vi "Cmd.Trigger.vi"(6 "Timeout [ms] (1000)":i32=1000, 8 "error in":errorcluster, 10 "TriggerNo":T1 items=["1"=1, "2"=2, "3"=3, "4"=4, "ALL"=5], 11 "cID in":refnum<k5>) -> (0 "error out":errorcluster, 1 "debug":string, 3 "cID out":refnum<k5>)   [LabVIEW 2016]
uses:
  controls/TriggerNo.ctl
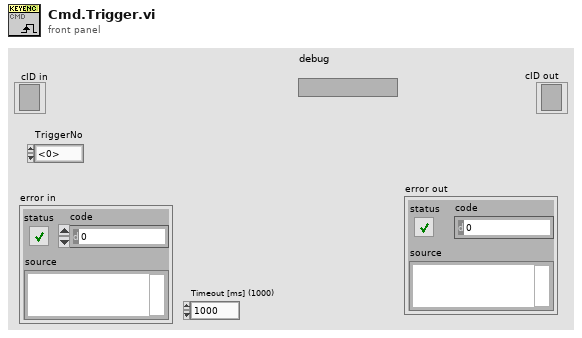
[diagram p1: front panel]
types:
  T1 = typedef "TriggerNo.ctl" = u8
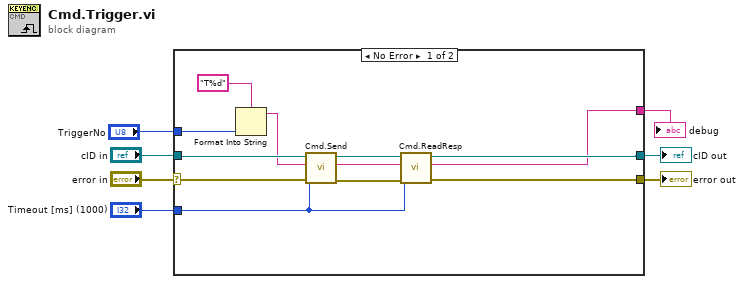
[diagram p0: block diagram]
diagram:
  n1 = case shown="No Error" "error in" {
    selector: "error in" -> [w17 w19]
    tunnel: "Timeout [ms] (1000)" -> [w11 _]
    tunnel: "cID in" -> [w18 w20]
    tunnel: [w10 w20] -> w4
    tunnel: [w9 w19] -> w3
    tunnel: "TriggerNo" -> [w16 _]
    tunnel: [w8 _] -> w1
    frame No Error {
      n2 = Format Into String(format string="T%d", w16) -> (resulting string=w13:string)  [unwired: 2 in, 1 out]
      n3 = call "Cmd.Send.vi"("error in (no error)"=w17, "Timeout [ms] (1000)"=w11, "Command"=w13, "connection ID"=w18) -> ("error out"=w12:errorcluster, "connection ID out"=w14:refnum<k5>)  [unwired: 6 in]
      n4 = call "Cmd.ReadResp.vi"("error in (no error)"=w12, "Timeout [ms] (1000)"=w11, "Request"=w13, "connection ID"=w14) -> ("error out"=w9:errorcluster, "ResponseParameters"=w8:string, "connection ID out"=w10:refnum<k5>)  [unwired: 5 in]
    }
    frame Error {
    }
  }
  "cID out" <- w4
  "error out" <- w3
  "debug" <- w1
